vi "Configure Alarm Output Type.vi"(0 "VISA resource name":refnum<visa-resource-name>, 1 "Unit Address (1)":i16=1, 2 "Alarm Type (0: Off)":u16(ring) items=["Off", "Process", "Deviation"], 5 "Alarm Output (1)":i16=1, 7 "Name (ALARM1)":string="ALARM1", 9 "Alarm Source (0: Input 1)":u16(ring) items=["Input 1", "Input 2", "Input 3"], 11 "error in (no error)":errorcluster {"code" format="%.0x"}) -> (4 "VISA resource name out":refnum<visa-resource-name>, 15 "error out":errorcluster {"code" format="%.0x"})   [LabVIEW 2010]
doc: "This VI configures alarm type and alarm source."
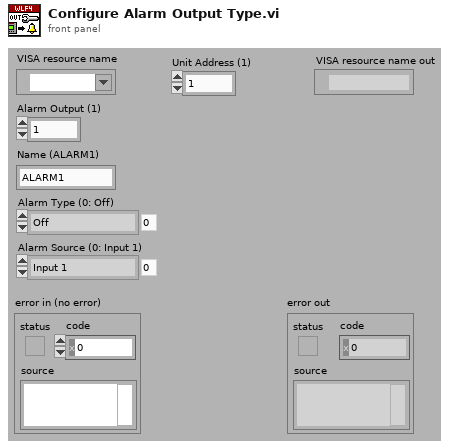
[diagram p1: front panel]
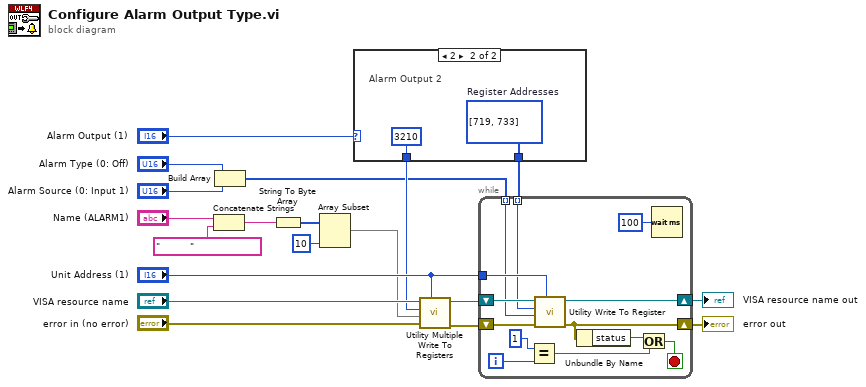
[diagram p0: block diagram]
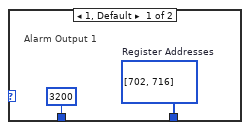
[diagram p2: hidden frame]
diagram:
  n1 = Concatenate Strings("Name (ALARM1)", "          " ("string")) -> (w7:string)
  n2 = Build Array("Alarm Type (0: Off)", "Alarm Source (0: Input 1)") -> (w1:u16[])
  n3 = String To Byte Array(string=w7) -> (unsigned byte array=w8:u8[])
  n4 = Array Subset(array=w8, length=10) -> (w6:u8[])  [unwired: 1 in]
  n5 = case shown="2" "Alarm Output (1)" {
    tunnel: [w21 w23] -> w16
    tunnel: [3200 3210] -> w10
    frame 1, Default {
      w21 = i32[] [702, 716]  # Register Addresses
      # "Alarm Output 1"
    }
    frame 2 {
      w23 = i32[] [719, 733]  # Register Addresses
      # "Alarm Output 2"
    }
  }
  n6 = call "Utility Multiple Write To Registers.vi"("Unit Address (1)"="Unit Address (1)", "error in (no error)"="error in (no error)", "Array Of Data"=w6, "Register Address (0)"=w10, "VISA resource name"="VISA resource name") -> ("error out"=w14:errorcluster, "VISA resource name out"=w12:refnum<visa-resource-name>)  [unwired: 5 in]
  n7 = while {
    tunnel: "Unit Address (1)" -> [w36]
    shift-right: [w33] -> w19
    shift-left: w12 -> [w35]
    shift-right: [w29] -> w18
    shift-left: w14 -> [w34]
    tunnel: w16 -> [w31] mode=indexing
    tunnel: w1 -> [w30] mode=indexing
    i -> [w25]
    stop <- w27 stop-if-true
    n8 = Equal?(x=1, y=w25) -> (x = y?=w24:bool)
    n9 = call "Utility Write To Register.vi"("Unit Address (1)"=w36, "error in (no error)"=w34, "Data (0)"=w30, "Register Address (0)"=w31, "VISA resource name"=w35) -> ("error out"=w29:errorcluster, "VISA resource name out"=w33:refnum<visa-resource-name>)  [unwired: 5 in]
    n10 = Unbundle By Name(w29) -> ("status"=w28:bool)
    n11 = Or(x=w28, y=w24) -> (x .or. y?=w27:bool)
    n12 = Wait (ms)(milliseconds to wait=u32 100) -> ()  [unwired: 1 out]
  }
  "error out" <- w18
  "VISA resource name out" <- w19
